vi "Create-Order.vi"(6 "# of Shares":u32, 7 "OrderRefNum":u64, 9 "Price":dbl, 10 "Operation":enum16{"GetAll", "AddOrder", "DeleteOrder"}(ring), 11 "Side":enum16{"Buy", "Sell"}(ring)) -> (3 "Array":u64[](array[numeric]))   [LabVIEW 2016]
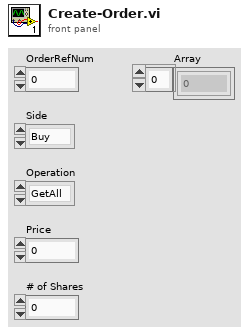
[diagram p1: front panel]
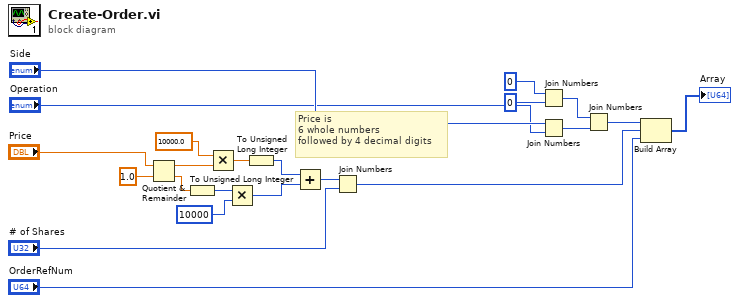
[diagram p0: block diagram]
diagram:
  # "Price is\n6 whole numbers\nfollowed by 4 decimal digits"
  n1 = Quotient & Remainder(x="Price", y=1.0) -> (x-y*floor(x/y)=w12:dbl, floor(x/y)=w13:dbl)
  n2 = To Unsigned Long Integer(number=w13) -> (unsigned 32bit integer=w18:u32)
  n3 = Multiply(x=10000.0, y=w12) -> (x*y=w14:dbl)
  n4 = Multiply(x=w18, y=u32 10000 ("x")) -> (x*y=w17:u32)
  n5 = To Unsigned Long Integer(number=w14) -> (unsigned 32bit integer=w16:u32)
  n6 = Add(x=w16, y=w17) -> (x+y=w20:u32)
  n7 = Join Numbers(hi=w20, lo="# of Shares") -> ((hi.lo)=w21:u64)
  n8 = Join Numbers(hi=u16 0, lo=u16 0) -> ((hi.lo)=w5:u32)
  n9 = Join Numbers(hi="Side", lo="Operation") -> ((hi.lo)=w3:u32)
  n10 = Join Numbers(hi=w5, lo=w3) -> ((hi.lo)=w4:u64)
  n11 = Build Array(w4, w21, "OrderRefNum") -> (→"Array":u64[])
